vi "Update.vi"(11 "Core Data in":T1) -> (2 "Screen":picture, 3 "Core Data out":T1)   [LabVIEW 2020, in "Amnesia.lvlib"]
uses:
  Amnesia.lvlib
  Scene/Scene.lvclass
  Scene/Scene.lvclass/Scene.ctl
  Core Data.ctl
  Scene/Mouse Button Held.ctl
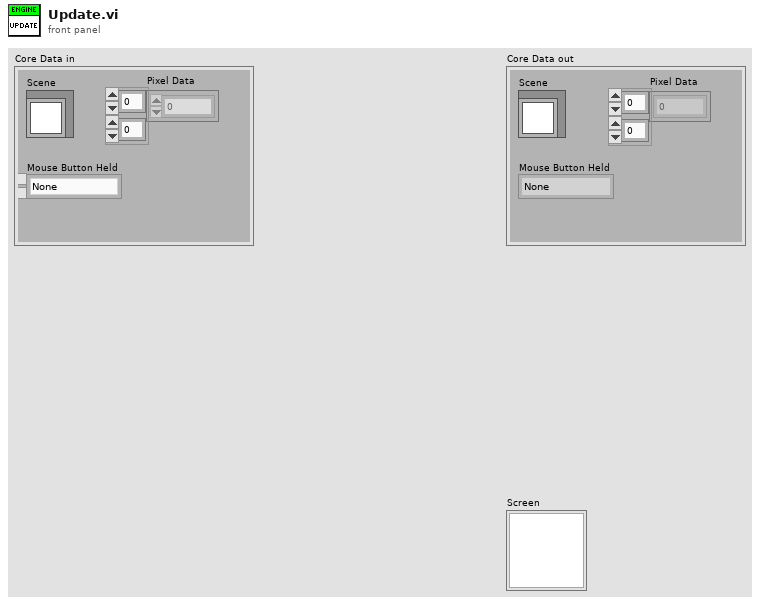
[diagram p1: front panel]
types:
  T1 = typedef "Amnesia.lvlib/Core Data.ctl" = cluster{"Pixel Data":u32[][], "Scene":refnum<class "Scene.lvclass">, "Mouse Button Held":T2}
  T2 = typedef "Scene.lvclass/Mouse Button Held.ctl" = enum16{"None", "Left", "Middle", "Right"}
  T3 = typedef "Scene.lvclass/Stats.ctl" = cluster{"Transform And Project Duration":dbl, "Raster Duration":dbl, "Present Duration":dbl, "Frame Rate":dbl, "Visible Triangles":i32, "Delta Time":dbl}
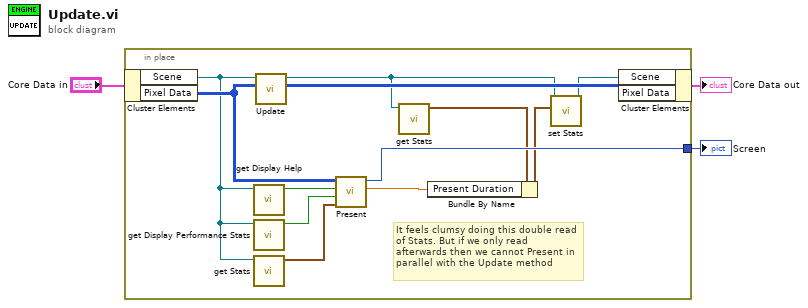
[diagram p0: block diagram]
diagram:
  n1 = in-place {
    in-place-border: [w13] -> w2
    # "It feels clumsy doing this double read of Stats. But if we only read afterwards then we cannot Present in parallel with the Update method"
    n2 = in-place-cluster #1("Core Data in") -> ("Scene"=w5:refnum<class "Scene.lvclass">, "Pixel Data"=w14:u32[][])
    n3 = call "get Display Help.vi"("Scene in"=w5) -> ("Display Help"=w7:bool)  [unwired: 10 in]
    n4 = call "get Display Performance Stats.vi"("Scene in"=w5) -> ("Display Stats"=w6:bool)  [unwired: 10 in]
    n5 = call "get Stats.vi"("Scene in"=w5) -> ("Stats"=w4:T3)  [unwired: 10 in]
    n6 = call "Update.vi"("Pixel Data in"=w14, "Scene in"=w5) -> ("Pixel Data out"=w15:u32[][], "Scene out"=w11:refnum<class "Scene.lvclass">)  [unwired: 8 in]
    n7 = call "Present.vi"("Stats"=w4, "Display Stats"=w6, "Display Help"=w7, "Pixel Data"=w14) -> ("Present Duration [s]"=w9:dbl, "2D Picture"=w13:picture)  [unwired: 6 in]
    n8 = call "get Stats.vi"("Scene in"=w11) -> ("Stats"=w10:T3)  [unwired: 10 in]
    n9 = Bundle By Name(cluster=w10, "Present Duration"=w9) -> (w8:T3)
    n10 = call "set Stats.vi"("Stats"=w8, "Scene in"=w11) -> ("Scene out"=w12:refnum<class "Scene.lvclass">)  [unwired: 9 in]
    n11 = in-place-cluster #1("Scene"=w12, "Pixel Data"=w15) -> (→"Core Data out":T1)
  }
  "Screen" <- w2
